vi "Write_CmdSingleParam_Wrapper.vi"(8 "error in (no error)":errorcluster, 11 "Multiplexer_Opmux in":refnum<class "Multiplexer_Opmux.lvclass">) -> (0 "error out":errorcluster, 3 "Multiplexer_Opmux out":refnum<class "Multiplexer_Opmux.lvclass">)   [LabVIEW 2014, in "Multiplexer_Opmux.lvclass"]
uses:
  Multiplexer_Opmux.lvclass
  CommandsEnum.ctl
panel:
  in  "CMD":T1
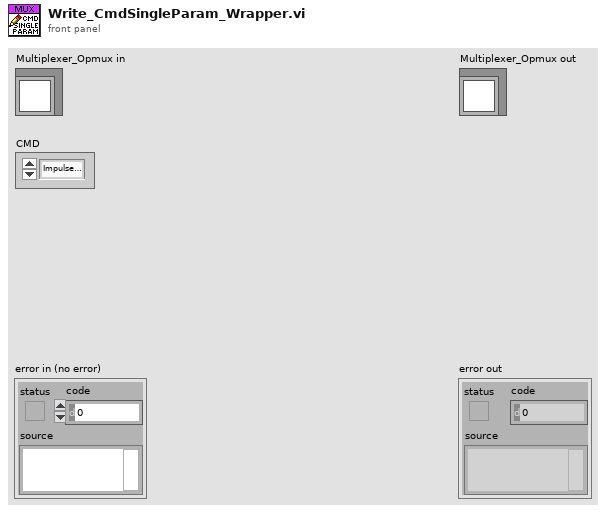
[diagram p1: front panel]
types:
  T1 = typedef "CommandsEnum.ctl" = enum16{"Impulse Voltage", "Table"}
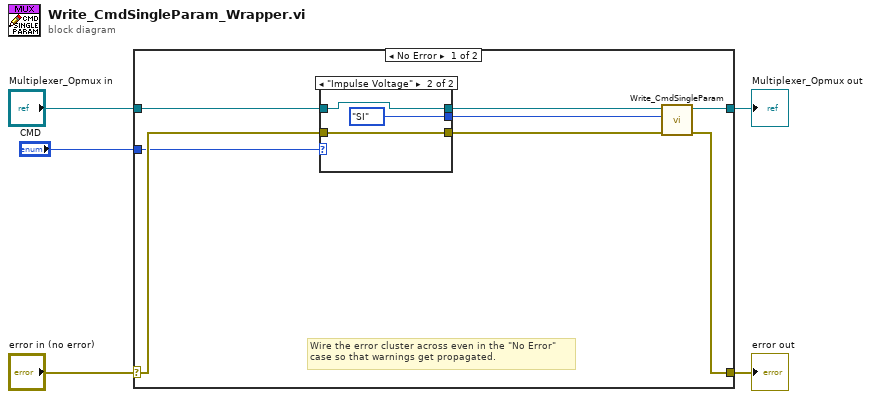
[diagram p0: block diagram]
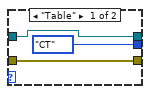
[diagram p2: hidden frame]
diagram:
  n1 = case shown="No Error" "error in (no error)" {
    selector: "error in (no error)" -> [w12 w21]
    tunnel: [w8 w21] -> w4
    tunnel: [w7 w20] -> w2
    tunnel: "Multiplexer_Opmux in" -> [w13 w20]
    tunnel: "CMD" -> [w11 _]
    frame No Error {
      # "Wire the error cluster across even in the \"No Error\"\ncase so that warnings get propagated."
      n2 = case shown="\"Impulse Voltage\"" w11 {
        tunnel: w13 -> [w15 w18]
        tunnel: [w15 w18] -> w10
        tunnel: [w14 w17] -> w9
        tunnel: w12 -> [w14 w17]
        tunnel: [enum16{"SA", "GT", "SI", "SL", "ST", "CT"}."CT" ("Command") enum16{"SA", "GT", "SI", "SL", "ST", "CT"}."SI" ("Command")] -> w6
        frame "Table" {
        }
        frame "Impulse Voltage" {
        }
      }
      n3 = call-dynamic "Write_CmdSingleParam.vi"("error in (no error)"=w9, "Command"=w6, "Multiplexer_Opmux in"=w10) -> ("error out"=w8:errorcluster, "Multiplexer_Opmux out"=w7:refnum<class "Multiplexer_Opmux.lvclass">)  [unwired: 7 in]
    }
    frame Error {
    }
  }
  "error out" <- w4
  "Multiplexer_Opmux out" <- w2
